vi "Configure PWM Task.vi"(8 "error in (no error)":errorcluster, 11 "DAQ Tasks":T1) -> (0 "error out":errorcluster, 3 "DAQ Tasks Out":T1)   [LabVIEW 2015]
doc: "Configure PWM Task by setting timing to implicit, and starting the task."
uses:
  DAQ Tasks.ctl
  <vilib>/DAQmx/configure/timing.llb/DAQmx Timing (Implicit).vi
  <resource>/objmgr/daqmx.rc
  DAQmx Module Runtime.lvclass
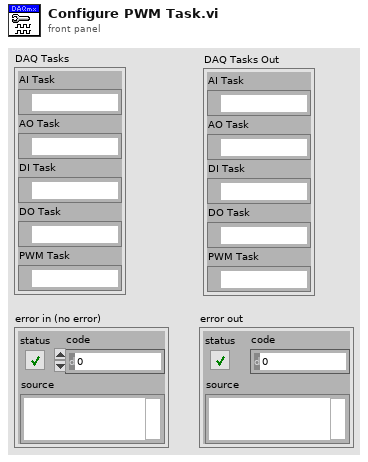
[diagram p1: front panel]
types:
  T1 = typedef "DAQmx Module Runtime.lvclass/DAQ Tasks.ctl" = cluster{"AI Task":refnum<k21>, "AO Task":refnum<k21>, "DI Task":refnum<k21>, "DO Task":refnum<k21>, "PWM Task":refnum<k21>}
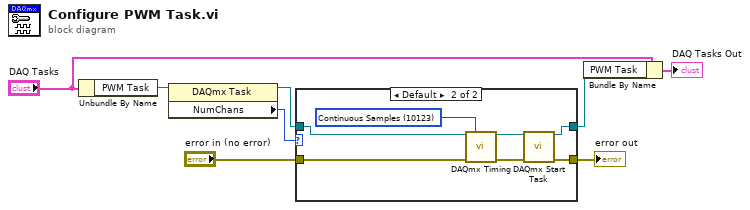
[diagram p0: block diagram]
diagram:
  n1 = Unbundle By Name("DAQ Tasks") -> ("PWM Task"=w6:refnum<k21>)
  n2 = property class="DAQmx Task"(reference=w6) -> (reference out=w7:refnum<k21>, "NumChans"=w8:u32)  [unwired: 1 in, 1 out]
  n3 = case shown="Default" w8 {
    tunnel: "error in (no error)" -> [w10 w15]
    tunnel: [w10 w13] -> w5
    tunnel: w7 -> [w9 w12]
    tunnel: [w9 w11] -> w3
    frame 0 {
      # "Don't start PWM task \nif there are no chans"
    }
    frame Default {
      w17 = 10123 items=["Finite Samples"=10178, "Continuous Samples"=10123, "Hardware Timed Single Point"=12522] ("sample mode")
      n4 = call-poly <vilib>:"DAQmx Timing.vi"("task/channels in"=w12, "sample mode"=w17, "error in"=w15) -> ("task out"=w16:refnum<k21>, "error out"=w14:errorcluster)  [unwired: 11 in]
      n5 = call <vilib>:"DAQmx Start Task.vi"("task/channels in"=w16, "error in"=w14) -> ("task out"=w11:refnum<k21>, "error out"=w13:errorcluster)  [unwired: 12 in]
    }
  }
  "error out" <- w5
  n6 = Bundle By Name(cluster="DAQ Tasks", "PWM Task"=w3) -> (→"DAQ Tasks Out":T1)
